vi "Process.vi"(0 "reference in":refnum<class "ZeroMQ.lvclass">, 5 "error in (no error)":errorcluster) -> (14 "reference out":refnum<class "ZeroMQ.lvclass">, 19 "error out":errorcluster)   [LabVIEW 2018, in "ZeroMQ.lvclass"]
uses:
  ZeroMQ.lvclass
  <vilib>/addons/zeromq/zmq_context.lvclass
  <vilib>/addons/zeromq/zmq_socket.lvclass
  <vilib>/addons/zeromq/socket_type.ctl
  <vilib>/Utility/SystemLogging/NI_SystemLogging.lvlib
  <vilib>/addons/zeromq/zeromq.lvlib
panel:
  out "Read Error":errorcluster
  out "Process Error":errorcluster
  out "Lib path":path
  out "Waveform Chart":u32(graph)
  out "LastExectime":u32
  out "Connection String":string
  out "Output":string
  out "Input":string
  out "Message counter":i32
  out "Last Command":string
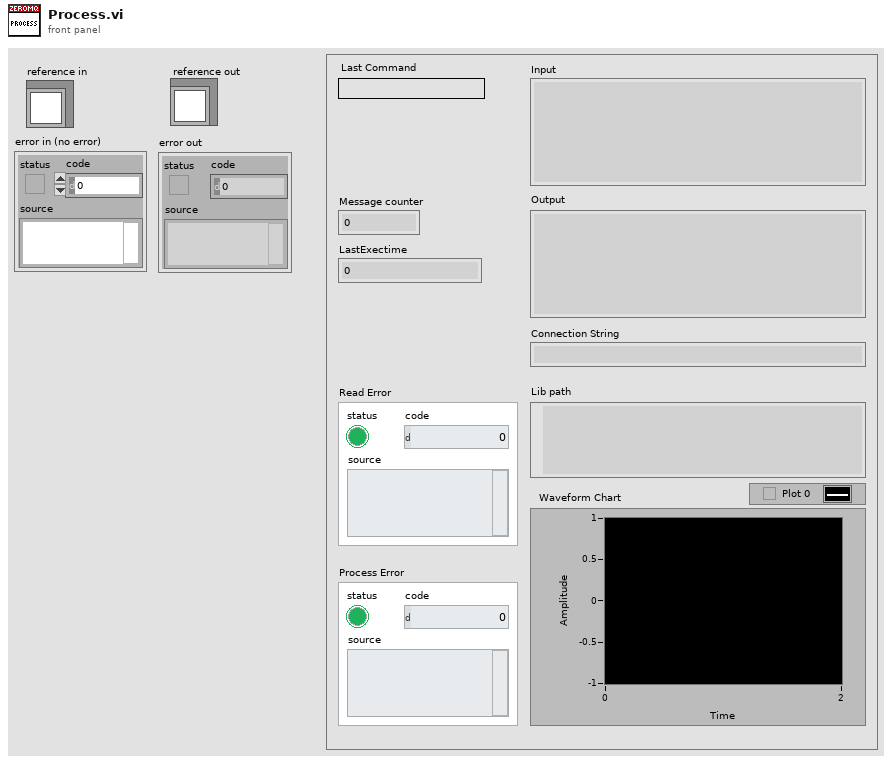
[diagram p1: front panel]
types:
  T1 = cluster{"Core":cluster{"This VI":refnum<vi>, "Timeout":i32, "Events":cluster{"EventsToProcess":refnum<event-registration>}, "EventFromProcess":refnum<user-event>, "ProcessSyncQueue":refnum<queue>, "QueueFromProcess":refnum<queue>, "Command":string, "Data":variant}, "0MQ":refnum<class "zmq_context.lvclass">, "Socket":refnum<class "zmq_socket.lvclass">}
  T2 = typedef "zeromq.lvlib/socket_type.ctl" = enum8{"ZMQ_PAIR", "ZMQ_PUB", "ZMQ_SUB", "ZMQ_REQ", "ZMQ_REP", "ZMQ_DEALER", "ZMQ_ROUTER", "ZMQ_PULL", "ZMQ_PUSH", "ZMQ_XPUB", "ZMQ_XSUB", "ZMQ_STREAM", "ZMQ_SERVER", "ZMQ_CLIENT", "ZMQ_RADIO", "ZMQ_DISH", "ZMQ_GATHER", "ZMQ_SCATTER", "ZMQ_DGRAM"}
  T3 = enum32{"Invalid", "Standard", "Closed", "Hidden", "Minimized", "Maximized"}
  T4 = cluster{"EventsToProcess":refnum<event-registration>}
  T5 = enum16{"Core Data", "Active Object", "UI: Initialize", "AO: Started"}[]
  T6 = typedef "ZeroMQ.lvclass/ObjectAttributes.ctl" = cluster{"IP":string, "Port":string}
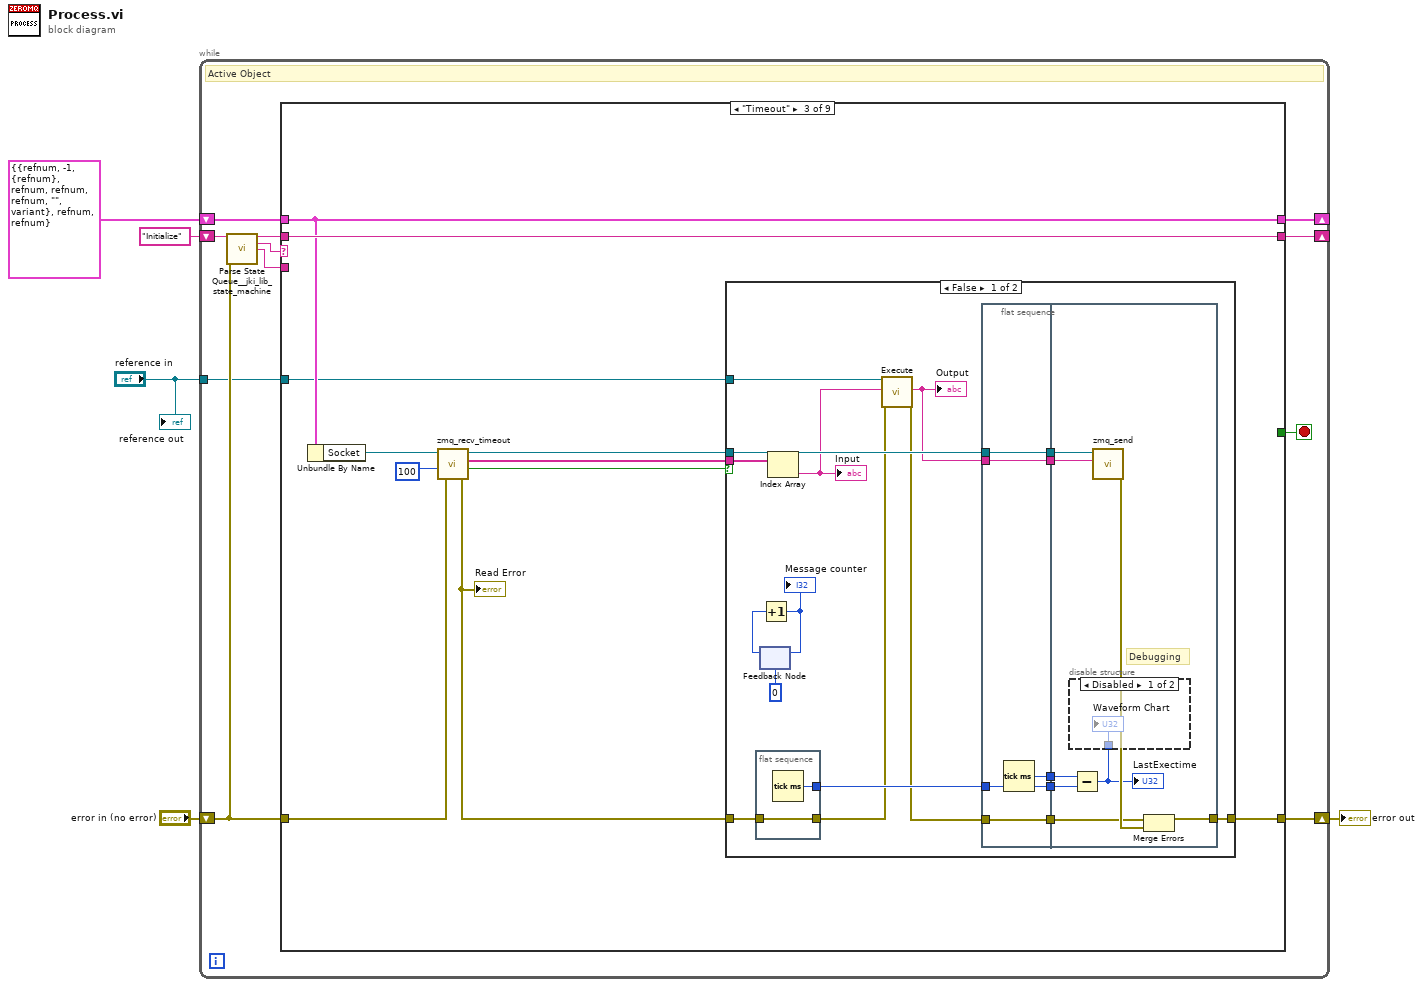
[diagram p0: block diagram]
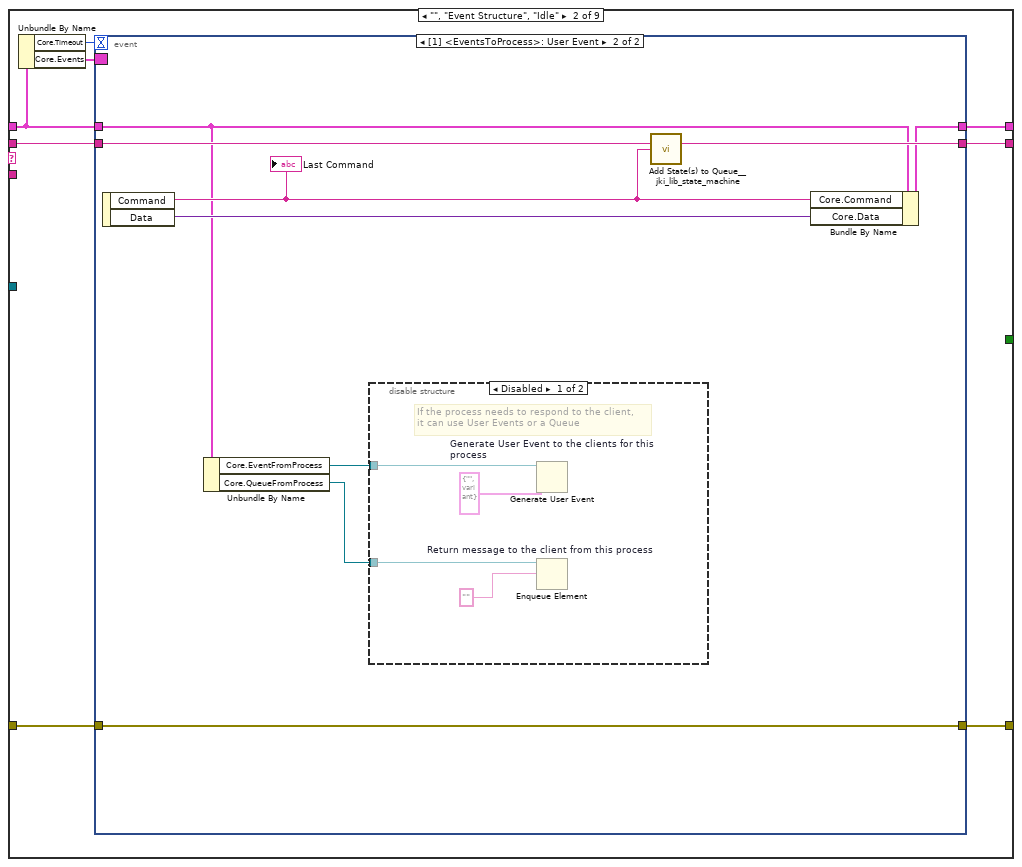
[diagram p3: hidden frame]
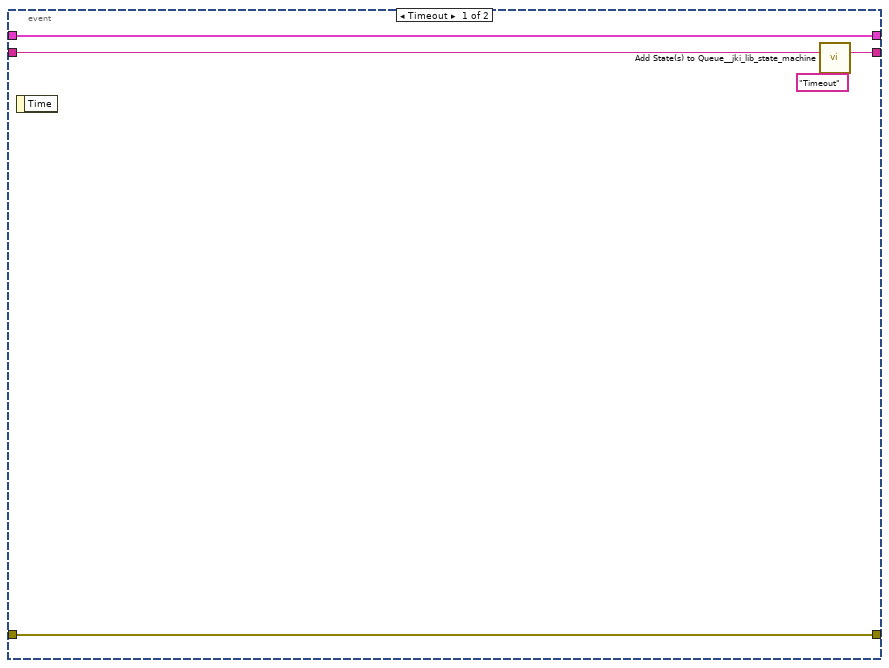
[diagram p4: hidden frame]
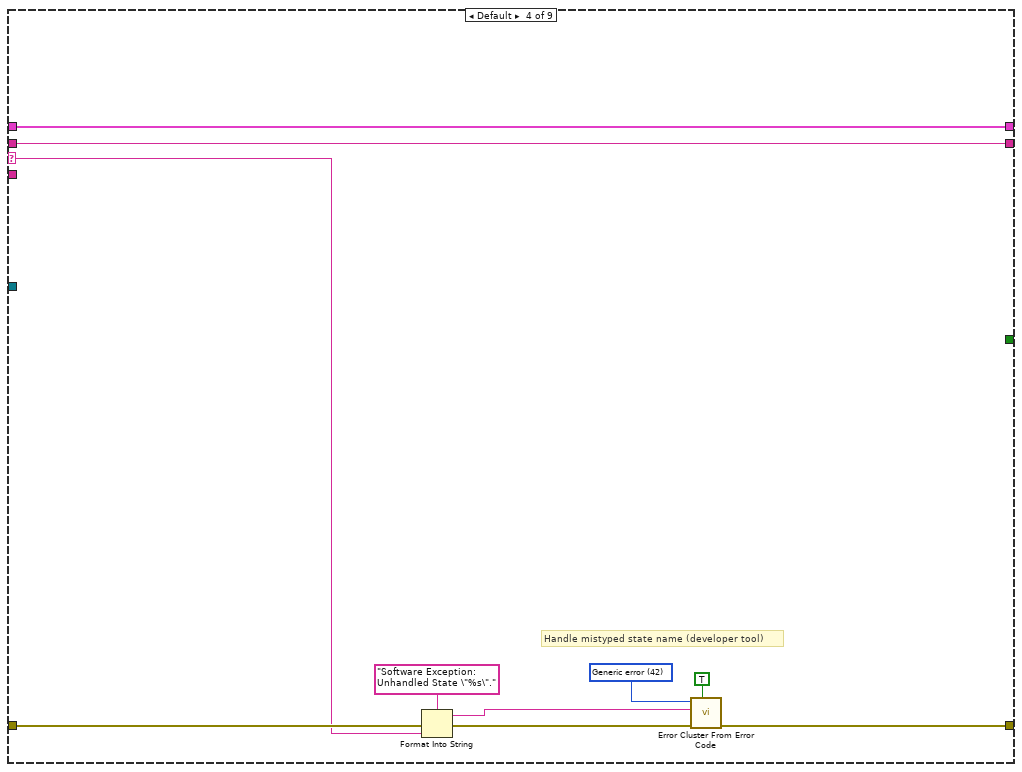
[diagram p8: hidden frame]
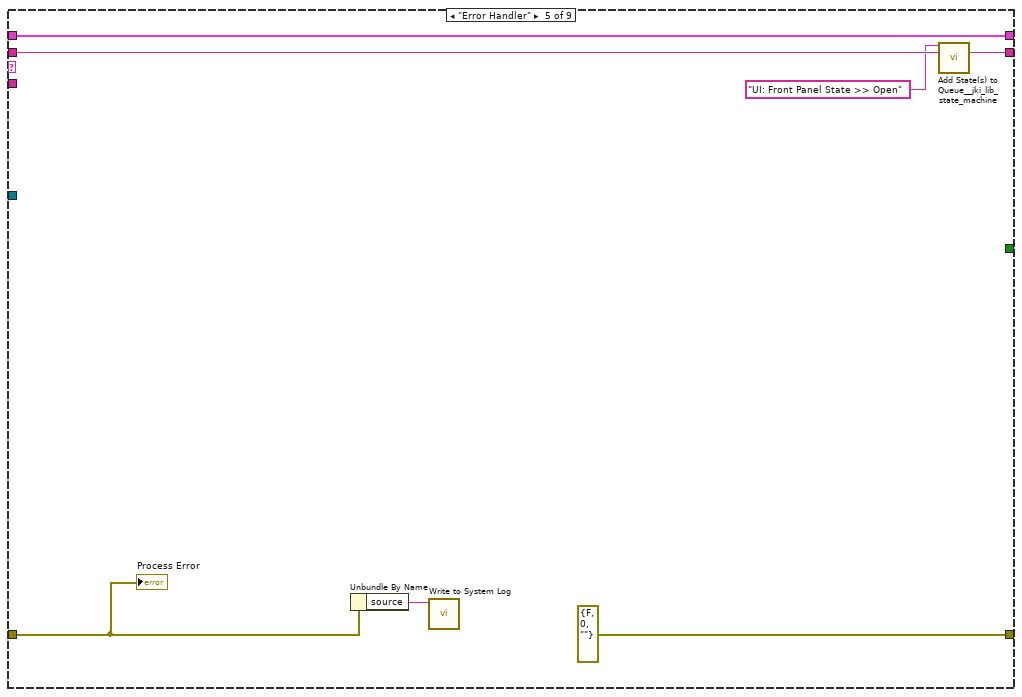
[diagram p9: hidden frame]
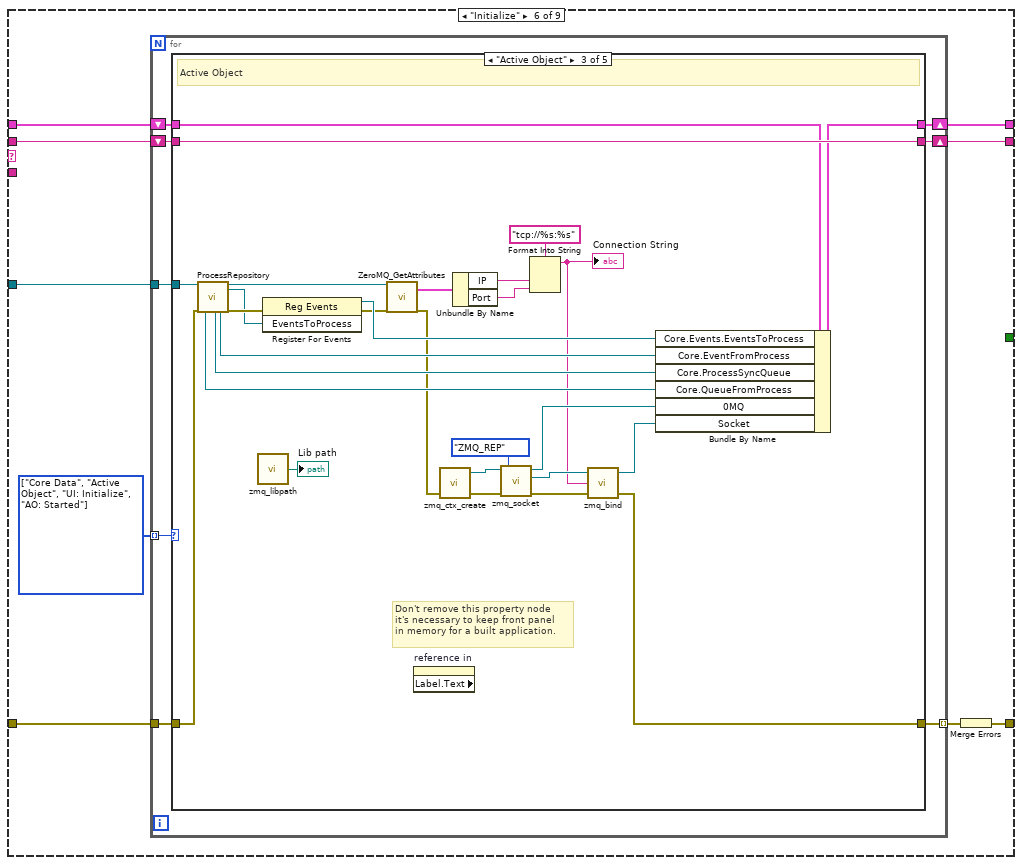
[diagram p10: hidden frame]
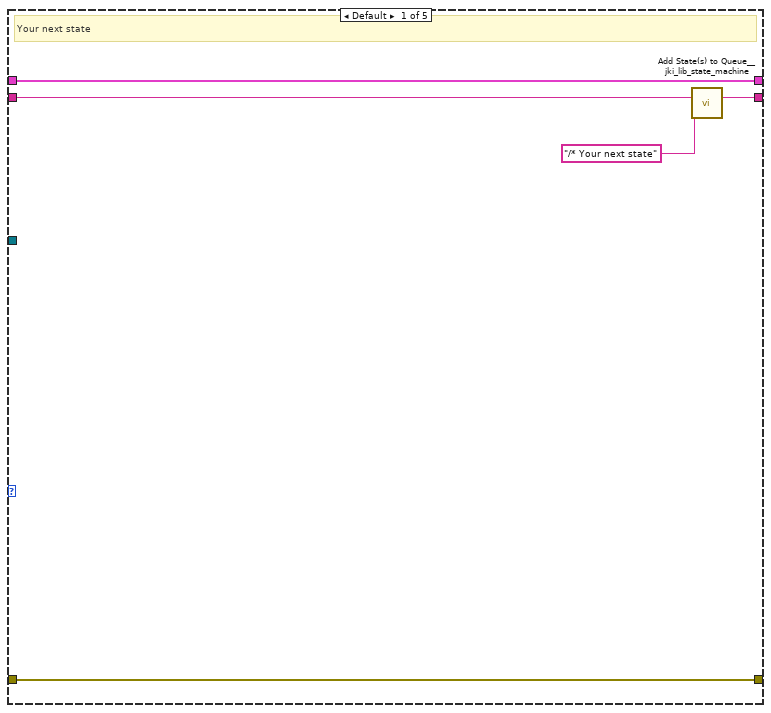
[diagram p11: hidden frame]
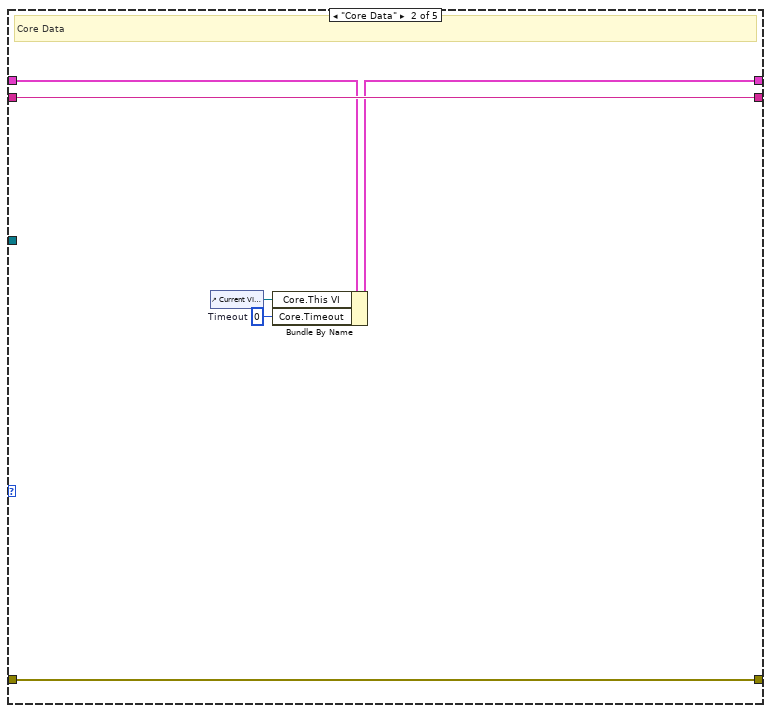
[diagram p12: hidden frame]
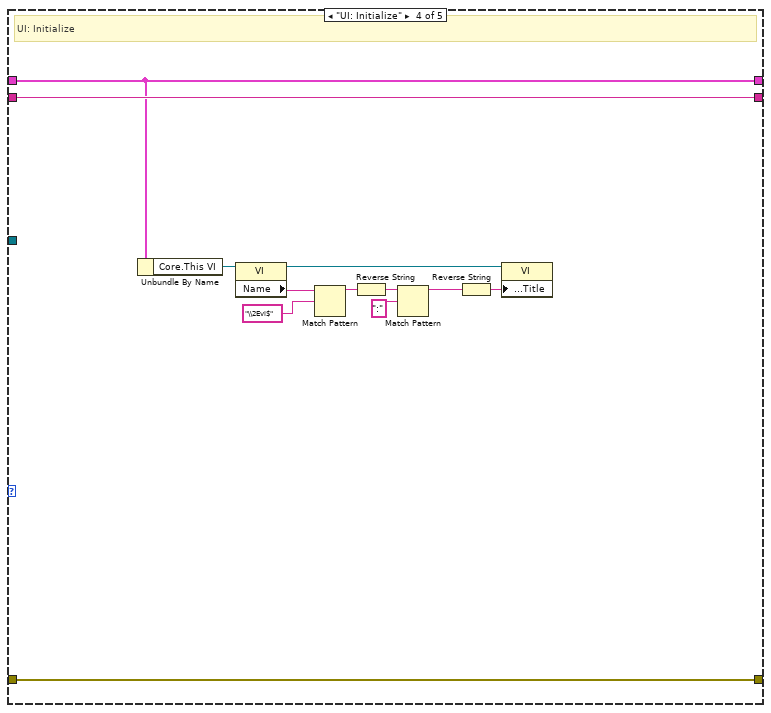
[diagram p13: hidden frame]
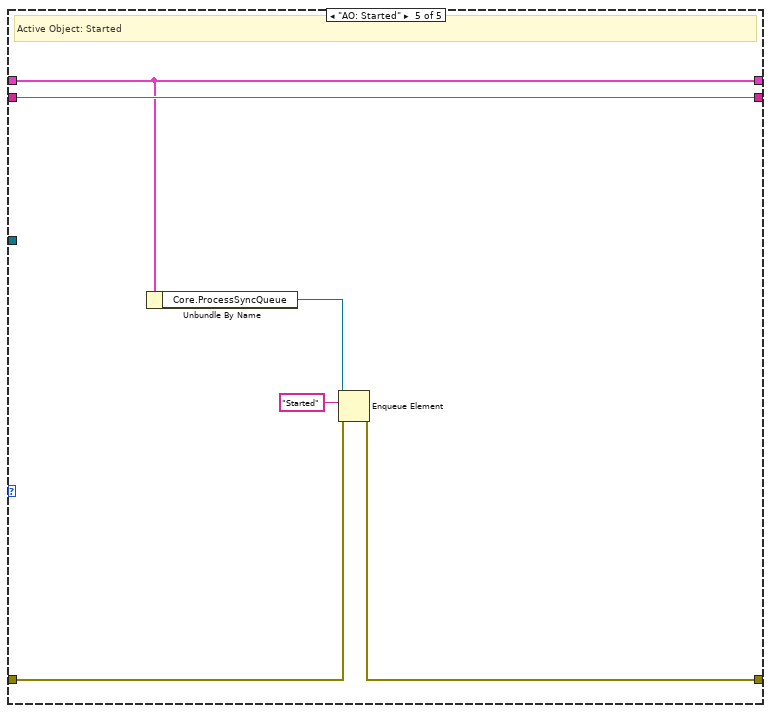
[diagram p14: hidden frame]
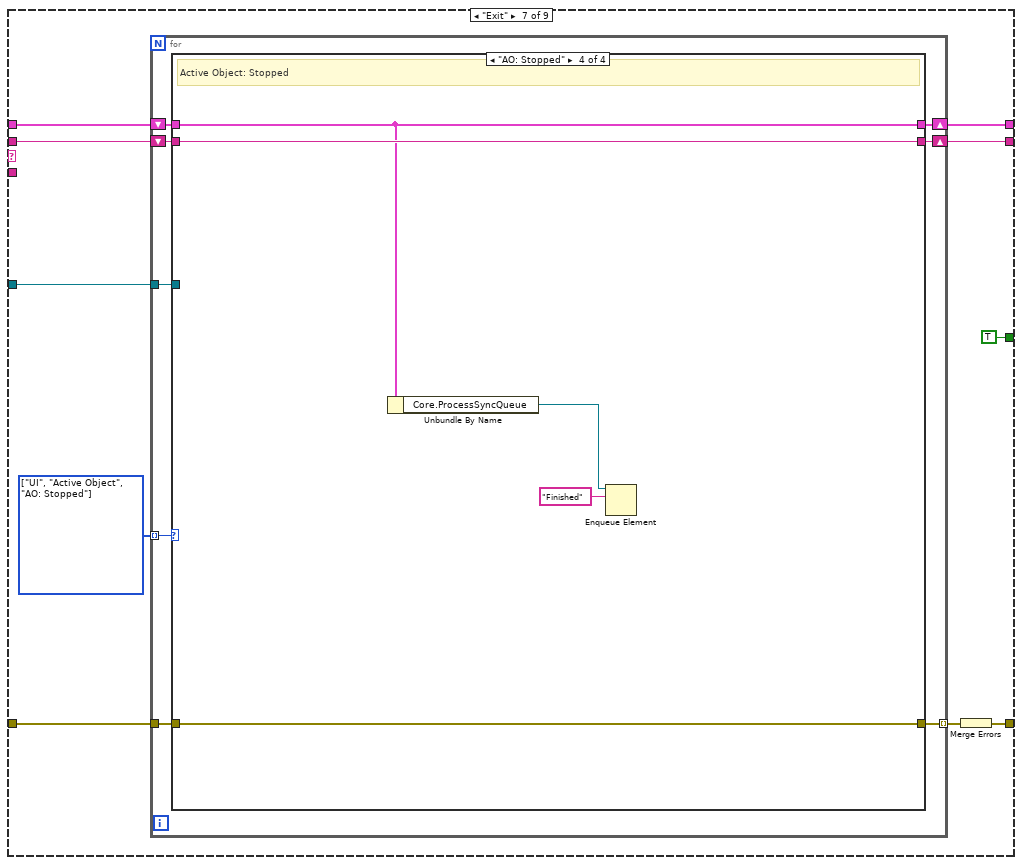
[diagram p15: hidden frame]
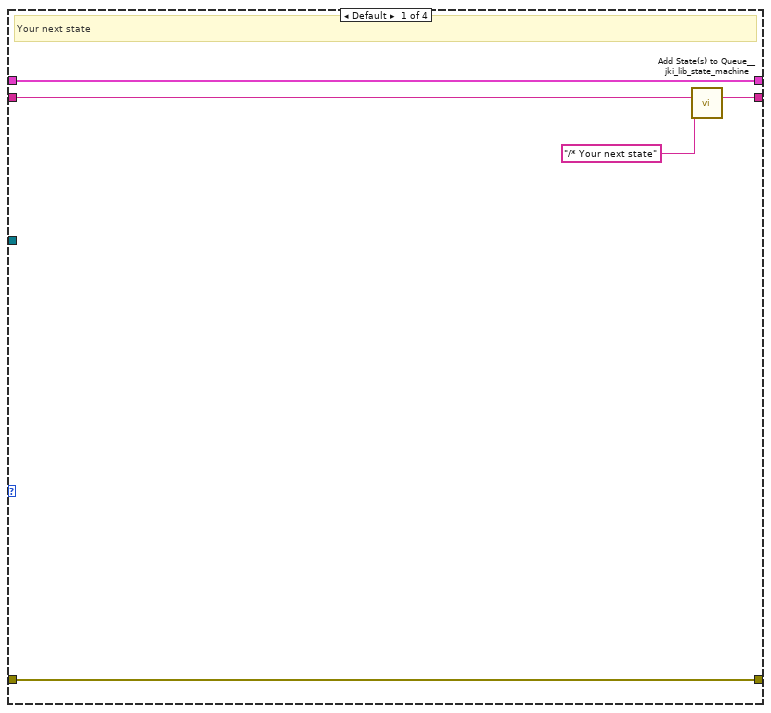
[diagram p16: hidden frame]
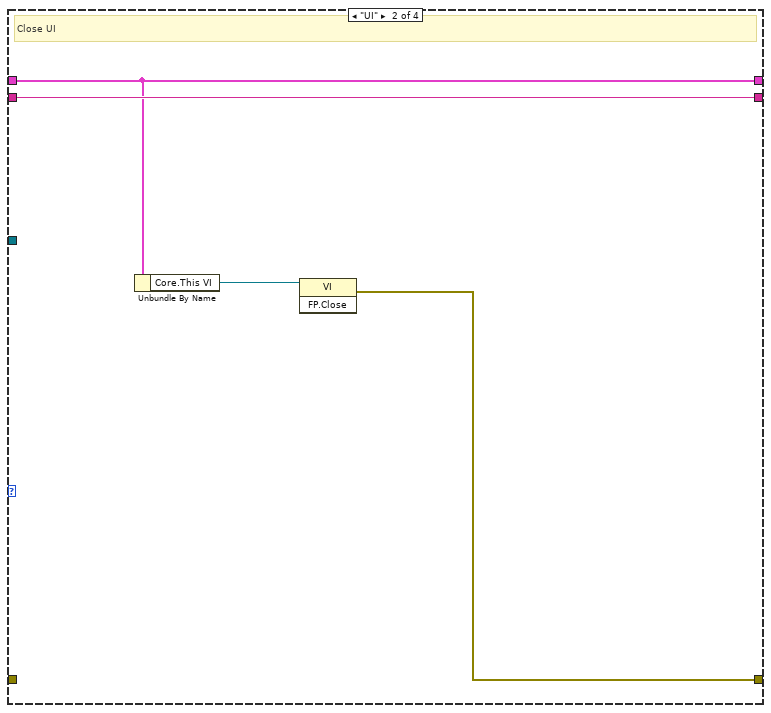
[diagram p17: hidden frame]
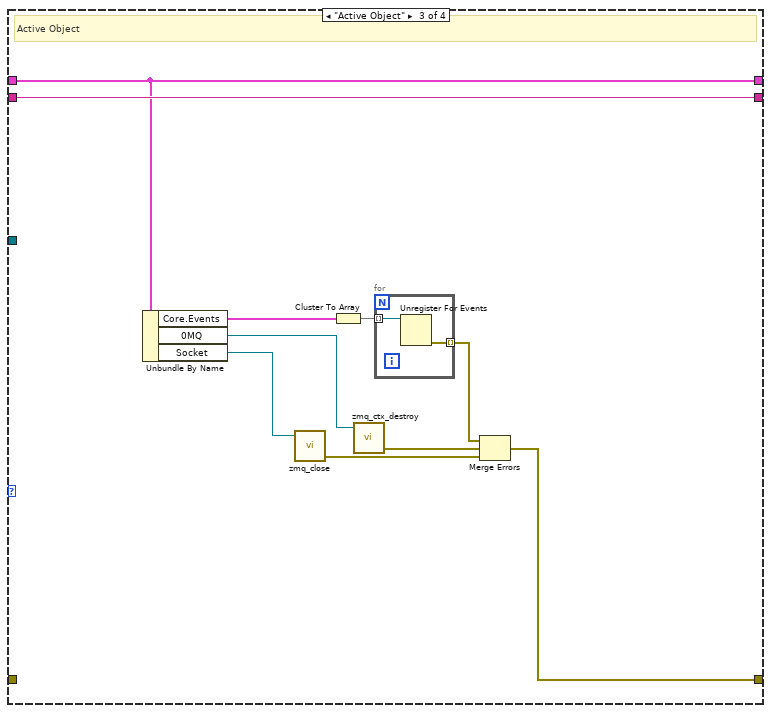
[diagram p18: hidden frame]
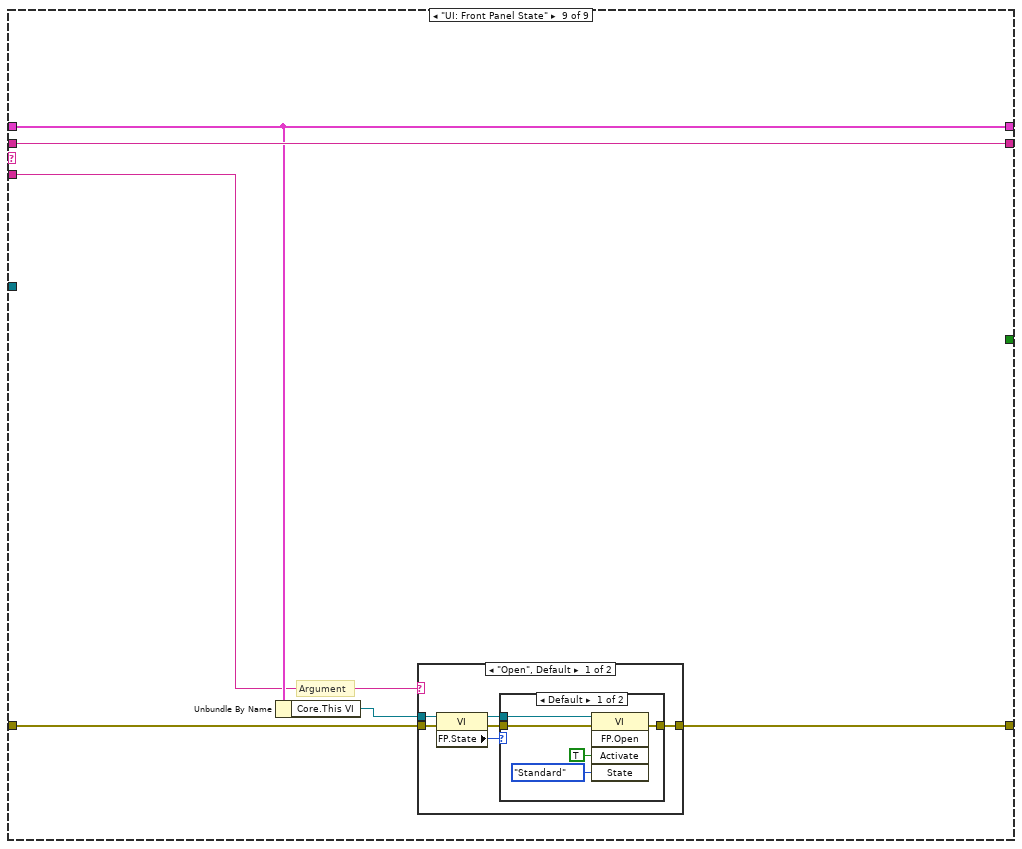
[diagram p20: hidden frame]
diagram:
  n1 = while {
    shift-right: [w15] -> w4
    shift-left: "error in (no error)" -> [w16]
    shift-right: [w8] -> _
    shift-left: "Initialize" ("States Out") -> [w11]
    shift-right: [w14] -> _
    shift-left: T1 {"Core"={"This VI"=refnum, "Timeout"=-1, "Events"={"EventsToProcess"=refnum}, "EventFromProcess"=refnum, "ProcessSyncQueue"=refnum, "QueueFromProcess"=refnum, "Command"="", "Data"=variant}, "0MQ"=refnum, "Socket"=refnum} ("LocalVariables") -> [w13]
    tunnel: "reference in" -> [w6]
    stop <- w7 stop-if-true
    # "Active Object"
    n2 = call <vilib>:"Parse State Queue__jki_lib_state_machine.vi"("State Queue"=w11, "Error In (no error)"=w16) -> ("Remaining States"=w10:string, "Current State"=w12:string, "Arguments"=w9:string)  [unwired: 11 in]
    n3 = case shown="\"Timeout\"" w12 {
      selector: w12 -> [_ _ _ w92 _ _ _ _ _]
      tunnel: w16 -> [w19 w21 w52 w94 w102 w113 w188 w229 w231]
      tunnel: [w19 w22 w53 w93 errorcluster {"status"=FALSE, "code"=0, "source"=""} ("error constant") w111 w186 w229 w230] -> w15
      tunnel: [w18 w27 w55 w101 w108 w115 w190 w228 w233] -> w14
      tunnel: w13 -> [w18 w23 w55 w101 w108 w114 w189 w228 w233]
      tunnel: w10 -> [w17 w25 w56 w100 w107 w116 w191 w227 w235]
      tunnel: w9 -> [_ _ _ _ _ _ _ _ w232]
      tunnel: [w17 w24 w56 w100 w106 w110 w185 w227 w235] -> w8
      tunnel: [_ _ _ _ _ _ TRUE _ _] -> w7
      tunnel: w6 -> [_ _ w51 _ _ w112 w187 _ _]
      frame "---------- Core ----------" {
      }
      frame "", "Event Structure", "Idle" {
        n4 = Unbundle By Name(w23) -> ("Core.Timeout"=w20:i32, "Core.Events"=w26:T4)
        n5 = event shown="[1] <EventsToProcess>: User Event" {
          selector: w26 -> [_ _]
          dyn-events: _ -> [_ _]
          timeout: w20 -> [_ _]
          tunnel: w23 -> [w32 w33]
          tunnel: [w32 w39] -> w27
          tunnel: [w30 w41] -> w24
          tunnel: w25 -> [w31 w40]
          tunnel: [w28 w34] -> w22
          tunnel: w21 -> [w28 w34]
          event Timeout {
            n6 = event-data() -> ()  [unwired: 1 in, 1 out]
            n7 = call <vilib>:"Add State(s) to Queue__jki_lib_state_machine.vi"("State(s) in (\"\")"=w31, "State(s) at Back (\"\")"="Timeout" ("State(s) at Back (\"\")")) -> ("States Out"=w30:string)  [unwired: 13 in]
          }
          event User Event {
            n8 = event-data() -> ("Command"=w35:string, "Data"=w38:variant)  [unwired: 1 in]
            "Last Command" <- w35
            n9 = Unbundle By Name(w33) -> ("Core.EventFromProcess"=w37:refnum<user-event>, "Core.QueueFromProcess"=w36:refnum<queue>)
            n10 = disable-structure shown="Disabled" {
              disable-tunnel: w37 -> [w45 _]
              disable-tunnel: w36 -> [w44 _]
              frame Disabled {
                # "If the process needs to respond to the client,\nit can use User Events or a Queue"
                n11 = Generate User Event "Generate User Event to the clients for this process"(user event=w45, event data cluster=cluster{"Command":string, "Data":variant} {"Command"="", "Data"=variant} ("event data")) -> ()  [unwired: 2 in, 2 out]
                n12 = Enqueue Element "Return message to the client from this process"(queue=w44, element="") -> ()  [unwired: 2 in, 3 out]
              }
              frame Enabled {
              }
            }
            n13 = call <vilib>:"Add State(s) to Queue__jki_lib_state_machine.vi"("State(s) in (\"\")"=w40, "State(s) at Back (\"\")"=w35) -> ("States Out"=w41:string)  [unwired: 13 in]
            n14 = Bundle By Name(cluster=w33, "Core.Command"=w35, "Core.Data"=w38) -> (w39:T1)
          }
        }
      }
      frame "Timeout" {
        n15 = Unbundle By Name(w55) -> ("Socket"=w48:refnum<class "zmq_socket.lvclass">)
        n16 = call <vilib>:"zmq_recv_timeout.vi"("error in"=w52, "timeout (ms)"=u32 100, "socket in"=w48) -> ("error out"=w47:errorcluster, "timeout?"=w49:bool, "parts"=w54:string[], "socket out"=w50:refnum<class "zmq_socket.lvclass">)  [unwired: 1 in]
        "Read Error" <- w47
        n17 = case shown="False" w49 {
          tunnel: [w72 w91] -> w53
          tunnel: w47 -> [w64 w91]
          tunnel: w54 -> [w61 _]
          tunnel: w51 -> [w74 _]
          tunnel: w50 -> [w70 _]
          frame False {
            n18 = flat-sequence {
              tunnel: [w76] -> w62
              tunnel: w64 -> [w76]
              tunnel: [w75] -> w65
              frame #0 {
                n19 = Tick Count (ms)() -> (millisecond timer value=w75:u32)
              }
            }
            n20 = feedback #1(0) -> (w59:i32)
            n21 = Increment(x=w59) -> (x+1=w58:i32)
            "Message counter" <- w58
            n22 = feedback-in #1(w58) -> ()
            n23 = Index Array(array=w61) -> (element=w60:string)  [unwired: 1 in]
            "Input" <- w60
            n24 = call-dynamic "Execute.vi"("reference in"=w74, "Input"=w60, "error in (no error)"=w62) -> ("Output"=w69:string, "error out"=w63:errorcluster)  [unwired: 14 in, 1 out]
            "Output" <- w69
            n25 = flat-sequence {
              tunnel: w63 -> [w81]
              tunnel: [w81] -> w73
              tunnel: [w80] -> w71
              tunnel: w70 -> [w80]
              tunnel: w69 -> [w79]
              tunnel: [w79] -> w68
              tunnel: [w78] -> w67
              tunnel: w65 -> [w77]
              tunnel: [w77] -> w66
              tunnel: w73 -> [w88]
              tunnel: [w87] -> w72
              tunnel: w71 -> [w86]
              tunnel: w68 -> [w85]
              tunnel: w67 -> [w84]
              tunnel: w66 -> [w83]
              frame #0 {
                n26 = Tick Count (ms)() -> (millisecond timer value=w78:u32)
              }
              frame #1 {
                # "Debugging"
                n27 = Subtract(x=w84, y=w83) -> (x-y=w82:u32)
                "LastExectime" <- w82
                n28 = disable-structure shown="Disabled" {
                  disable-tunnel: w82 -> [w90 _]
                  frame Disabled {
                    "Waveform Chart" <- w90
                  }
                  frame Enabled {
                  }
                }
                n29 = call <vilib>:"zmq_send.vi"("data"=w85, "socket in"=w86) -> ("error out"=w89:errorcluster)  [unwired: 5 in, 1 out]
                n30 = Merge Errors(w88, w89) -> (w87:errorcluster)
              }
            }
          }
          frame True {
          }
        }
      }
      frame Default {
        w98 = 42 items=["No error", "Argument error", "Memory is full", "Out of zone", "End of file", "File already open", "Generic file I/O error", "File not found", "File permission error", "Disk is full", "Duplicate path", "Too many files open", "System feature not enabled", "Resource file not found", "Cannot add resource", "Resource not found", "Image not found", "Image memory error", "Pen does not exist", "Config type invalid", "Config token not found", "Config parse error", "Config memory error", "Bad external code format", "Bad external code offset", "External code not present", "Null window", "Destroy window error", "Null menu", "Print aborted", "Bad print record", "Print driver error", "Windows error during printing", "Memory error during printing", "Print dialog error", "Generic print error", "Invalid device refnum", "Device not found", "Device parameter error", "Device unit error", "Cannot open device", "Device call aborted", "Generic error", "Cancelled by user", "Object ID too low", "Object ID too high", "Object not in heap", "Unknown heap", "Unknown object (invalid DefProc)", "Unknown object (DefProc not in table)", "Message out of range", "Invalid (null) method", "Unknown message", "Manager call not supported", "Bad address", "Network operation in progress", "Network operation timed out", "Connection is busy", "Network attribute not supported", "Network error", "Address in use", "System out of memory", "Connection aborted", "Connection refused", "Not connected", "Already connected", "Connection closed", "Initialization error (interapplication manager)", "Bad occurrence", "Wait on unbound occurrence handler", "Occurrence queue overflow", "Datalog type conflict", "Unused", "Unrecognized type (interapplication manager)", "Memory corrupt", "Failed to make temporary DLL", "Old CIN version", "Drag socket not found", "Failed to load drop-object", "Failed to register OLE object", "Failed to release OLE object", "Format specifier type mismatch", "Unknown format specifier", "Too few format specifiers", "Too many format specifiers", "Scan failed", "Newer CIN version", "Error converting to variant", "Runtime menu error", "Password tampered", "Variant attribute not found", "Incompatible variant data type", "Event data is not available", "Event Store is not present", "Occurrence is not found", "Event Queue is not created", "Event info is not available", "Refnum passed is NULL", "Error retrieving Class GUID", "Error retrieving CoClass GUID", "Error retrieving TypeLib GUID.", "Bad built application magic bytes.", "Specific driver is different from the specific driver associated with the Logical Name.", "There is no session opened to the class driver.", "Max Error", "MAX - Error with config objects", "MAX - Error loading configuration", "MAX - Group not supported"]
        # "Handle mistyped state name (developer tool)"
        n31 = Format Into String(format string="Software Exception: Unhandled State \"%s\"." ("message"), error in=w94, w92) -> (resulting string=w97:string, error out=w96:errorcluster)  [unwired: 1 in]
        n32 = call <vilib>:"Error Cluster From Error Code.vi"("show call chain? (False)"=TRUE, "error in (no error)"=w96, "error message (\"\")"=w97, "error code (0)"=w98) -> ("error out"=w93:errorcluster)  [unwired: 5 in]
      }
      frame "Error Handler" {
        n33 = Unbundle By Name(w102) -> ("source"=w104:string)
        n34 = call <vilib>:"Write to System Log.vi"("message"=w104) -> ()  [unwired: 10 in, 1 out]
        n35 = call <vilib>:"Add State(s) to Queue__jki_lib_state_machine.vi"("State(s) in Front (\"\")"="UI: Front Panel State >> Open" ("State(s) at Back (\"\")"), "State(s) in (\"\")"=w107) -> ("States Out"=w106:string)  [unwired: 13 in]
        "Process Error" <- w102
      }
      frame "Initialize" {
        w109 = T5 [enum."Core Data", enum."Active Object", enum."UI: Initialize", enum."AO: Started"] items=["Core Data", "Active Object", "UI: Initialize", "AO: Started"]
        n36 = for {
          tunnel: w113 -> [w124]
          tunnel: [w125] -> w117 mode=indexing
          tunnel: w112 -> [w119]
          shift-right: [w121] -> w115
          shift-left: w114 -> [w120]
          shift-right: [w123] -> w110
          shift-left: w116 -> [w122]
          tunnel: w109 -> [w118] mode=indexing
          n37 = case shown="\"Active Object\"" w118 {
            tunnel: [w130 w136 w141 w176 w177] -> w125
            tunnel: w124 -> [w130 w136 w155 w176 w178]
            tunnel: [w127 w135 w164 w175 w182] -> w123
            tunnel: w122 -> [w128 w135 w164 w175 w182]
            tunnel: [w129 w132 w156 w165 w179] -> w121
            tunnel: w120 -> [w129 w133 w157 w165 w179]
            tunnel: w119 -> [_ _ w154 _ _]
            frame Default {
              # "Your next state"
              n38 = call <vilib>:"Add State(s) to Queue__jki_lib_state_machine.vi"("State(s) in (\"\")"=w128, "State(s) at Back (\"\")"="/* Your next state" ("State(s) at Back (\"\")")) -> ("States Out"=w127:string)  [unwired: 13 in]
            }
            frame "Core Data" {
              w131 = 0  # Timeout
              # "Core Data"
              n39 = control-ref of="Current VI Reference"() -> (w134:refnum<vi>)
              n40 = Bundle By Name(cluster=w133, "Core.This VI"=w134, "Core.Timeout"=w131) -> (w132:T1)
            }
            frame "Active Object" {
              # "Don't remove this property node\nit's necessary to keep front panel\nin memory for a built application."
              # "Active Object"
              n41 = call "ProcessRepository.vi"("reference in"=w154, "error in (no error)"=w155) -> ("QueueFromProcess"=w158:refnum<queue>, "ProcessSyncQueue"=w159:refnum<queue>, "EventFromProcess"=w160:refnum<user-event>, "reference out"=w150:refnum<class "ZeroMQ.lvclass">, "EventsToProcess"=w162:refnum<user-event>, "error out"=w163:errorcluster)  [unwired: 10 in, 2 out]
              n42 = call <vilib>:"zmq_libpath.vi"() -> ("path"=→"Lib path":path)
              n43 = register-events(error in=w163, w162) -> (reference out=w161:refnum<event-registration>, error out=w149:errorcluster)  [unwired: 1 in]
              n44 = call "ZeroMQ_GetAttributes.vi"("reference in"=w150, "error in (no error)"=w149) -> ("Data"=w148:T6, "error out"=w137:errorcluster)  [unwired: 14 in, 2 out]
              n45 = property on="reference in" class="LVClassControl (strict)" props=["Label", "Text"]() -> ()  [unwired: 2 in, 3 out]
              n46 = call <vilib>:"zmq_ctx_create.vi"("error in"=w137) -> ("error out"=w138:errorcluster, "context out"=w153:refnum<class "zmq_context.lvclass">)  [unwired: 3 in]
              n47 = Unbundle By Name(w148) -> ("IP"=w143:string, "Port"=w140:string)
              n48 = call <vilib>:"zmq_socket.vi"("error in"=w138, "socket type"=socket_type."ZMQ_REP", "context in"=w153) -> ("error out"=w146:errorcluster, "socket out"=w147:refnum<class "zmq_socket.lvclass">, "context out"=w151:refnum<class "zmq_context.lvclass">)  [unwired: 2 in]
              n49 = Format Into String(format string="tcp://%s:%s" ("endpoint"), w143, w140) -> (resulting string=w142:string)  [unwired: 2 in, 1 out]
              "Connection String" <- w142
              n50 = call <vilib>:"zmq_bind.vi"("error in"=w146, "endpoint"=w142, "socket in"=w147) -> ("error out"=w141:errorcluster, "socket out"=w145:refnum<class "zmq_socket.lvclass">)  [unwired: 1 in]
              n51 = Bundle By Name(cluster=w157, "Core.Events.EventsToProcess"=w161, "Core.EventFromProcess"=w160, "Core.ProcessSyncQueue"=w159, "Core.QueueFromProcess"=w158, "0MQ"=w151, "Socket"=w145) -> (w156:T1)
            }
            frame "UI: Initialize" {
              # "UI: Initialize"
              n52 = Unbundle By Name(w165) -> ("Core.This VI"=w166:refnum<vi>)
              n53 = property class="VI"(reference=w166) -> (reference out=w167:refnum<vi>, "Name"=w174:string)  [unwired: 1 in, 1 out]
              n54 = Match Pattern(string=w174, regular expression="\\2Evi$") -> (before substring=w172:string)  [unwired: 1 in, 3 out]
              n55 = Reverse String(1:w172) -> (0:w171:string)
              n56 = Match Pattern(string=w171, regular expression=":") -> (before substring=w169:string)  [unwired: 1 in, 3 out]
              n57 = Reverse String(1:w169) -> (0:w168:string)
              n58 = property class="VI"(reference=w167, "Front Panel.Title"=w168) -> ()  [unwired: 1 in, 2 out]
            }
            frame "AO: Started" {
              # "Active Object: Started"
              n59 = Unbundle By Name(w179) -> ("Core.ProcessSyncQueue"=w180:refnum<queue>)
              n60 = Enqueue Element(queue=w180, element="Started", error in (no error)=w178) -> (error out=w177:errorcluster)  [unwired: 1 in, 2 out]
            }
          }
        }
        n61 = Merge Errors(w117) -> (w111:errorcluster)
      }
      frame "Exit" {
        w184 = enum16{"UI", "Active Object", "AO: Stopped"}[] [enum."UI", enum."Active Object", enum."AO: Stopped"] items=["UI", "Active Object", "AO: Stopped"]
        n62 = for {
          tunnel: w188 -> [w199]
          tunnel: [w200] -> w192 mode=indexing
          tunnel: w187 -> [w194]
          shift-right: [w196] -> w190
          shift-left: w189 -> [w195]
          shift-right: [w198] -> w185
          shift-left: w191 -> [w197]
          tunnel: w184 -> [w193] mode=indexing
          n63 = case shown="\"AO: Stopped\"" w193 {
            tunnel: [w205 w206 w214 w226] -> w200
            tunnel: w199 -> [w205 _ _ w226]
            tunnel: [w202 w209 w219 w225] -> w198
            tunnel: w197 -> [w203 w209 w219 w225]
            tunnel: [w204 w207 w215 w222] -> w196
            tunnel: w195 -> [w204 w207 w215 w222]
            tunnel: w194 -> [_ _ _ _]
            frame Default {
              # "Your next state"
              n64 = call <vilib>:"Add State(s) to Queue__jki_lib_state_machine.vi"("State(s) in (\"\")"=w203, "State(s) at Back (\"\")"="/* Your next state" ("State(s) at Back (\"\")")) -> ("States Out"=w202:string)  [unwired: 13 in]
            }
            frame "UI" {
              # "Close UI"
              n65 = Unbundle By Name(w207) -> ("Core.This VI"=w208:refnum<vi>)
              n66 = invoke class="VI" method="FP.Close"(reference=w208) -> (error out=w206:errorcluster)  [unwired: 2 in, 2 out]
            }
            frame "Active Object" {
              # "Active Object"
              n67 = Unbundle By Name(w215) -> ("Core.Events"=w218:T4, "0MQ"=w213:refnum<class "zmq_context.lvclass">, "Socket"=w212:refnum<class "zmq_socket.lvclass">)
              n68 = call <vilib>:"zmq_close.vi"("socket"=w212) -> ("error out"=w211:errorcluster)  [unwired: 4 in]
              n69 = Cluster To Array(cluster=w218) -> (array=w216:refnum<event-registration>[])
              n70 = call <vilib>:"zmq_ctx_destroy.vi"("context in"=w213) -> ("error out"=w210:errorcluster)  [unwired: 4 in]
              n71 = for {
                tunnel: w216 -> [w221] mode=indexing
                tunnel: [w220] -> w217 mode=indexing
                n72 = Unregister For Events(event registration refnum=w221) -> (error out=w220:errorcluster)  [unwired: 1 in]
              }
              n73 = Merge Errors(w217, w210, w211) -> (w214:errorcluster)
            }
            frame "AO: Stopped" {
              # "Active Object: Stopped"
              n74 = Unbundle By Name(w222) -> ("Core.ProcessSyncQueue"=w223:refnum<queue>)
              n75 = Enqueue Element(queue=w223, element="Finished") -> ()  [unwired: 2 in, 3 out]
            }
          }
        }
        n76 = Merge Errors(w192) -> (w186:errorcluster)
      }
      frame "---------- UI ----------" {
      }
      frame "UI: Front Panel State" {
        # "Argument"
        n77 = Unbundle By Name(w233) -> ("Core.This VI"=w234:refnum<vi>)
        n78 = case shown="\"Open\", Default" w232 {
          tunnel: w231 -> [w239 w249]
          tunnel: [w241 w253] -> w230
          tunnel: w234 -> [w240 w250]
          frame "Open", Default {
            n79 = property class="VI"(reference=w240, error in=w239) -> (reference out=w238:refnum<vi>, error out=w237:errorcluster, "FP.State"=w236:T3)
            n80 = case shown="Default" w236 {
              tunnel: [w244 w247] -> w241
              tunnel: w237 -> [w243 w247]
              tunnel: w238 -> [w242 _]
              frame Default {
                n81 = invoke class="VI" method="FP.Open"(reference=w242, error in=w243, "Activate"=TRUE, "State"=T3."Standard") -> (error out=w244:errorcluster)  [unwired: 1 in, 4 out]
              }
              frame "Standard" {
              }
            }
          }
          frame "Close" {
            n82 = property class="VI"(reference=w250, error in=w249) -> (reference out=w251:refnum<vi>, error out=w248:errorcluster, "FP.State"=w252:T3)
            n83 = case shown="\"Standard\"" w252 {
              tunnel: [w254 w257] -> w253
              tunnel: w248 -> [w254 w256]
              tunnel: w251 -> [_ w255]
              frame Default {
              }
              frame "Standard" {
                n84 = invoke class="VI" method="FP.Close"(reference=w255, error in=w256) -> (error out=w257:errorcluster)  [unwired: 1 in, 2 out]
              }
            }
          }
        }
      }
    }
  }
  "error out" <- w4
  "reference out" <- "reference in"
